vi "Validate Number.vi"(8 "error in (no error)":errorcluster, 11 "Number":i32 caption="Number to Validate") -> (0 "error out":errorcluster, 2 "Valid?":bool)   [LabVIEW 2017]
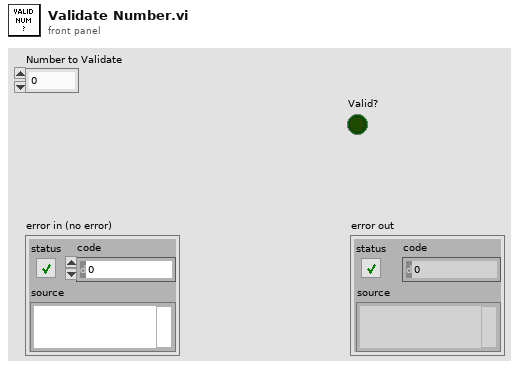
[diagram p1: front panel]
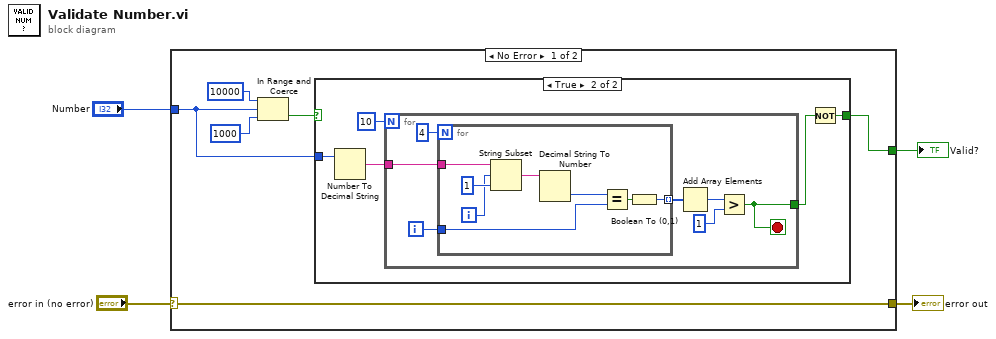
[diagram p0: block diagram]
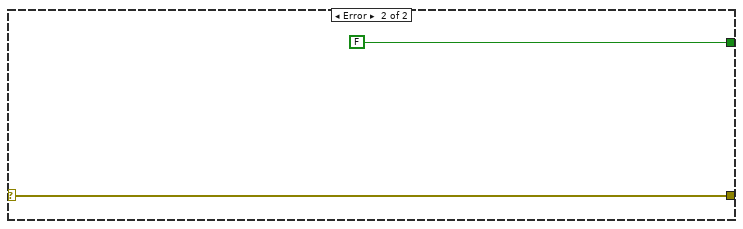
[diagram p3: hidden frame]
diagram:
  n1 = case shown="No Error" "error in (no error)" {
    selector: "error in (no error)" -> [w10 w33]
    tunnel: [w10 w33] -> w3
    tunnel: [w5 FALSE] -> w2
    tunnel: "Number" -> [w7 _]
    frame No Error {
      n2 = In Range and Coerce(upper limit=10000, x=w7, lower limit=1000) -> (In Range?=w6:bool)  [unwired: 1 out]
      n3 = case shown="True" w6 {
        selector: w6 -> [w11 _]
        tunnel: w7 -> [_ w16]
        tunnel: [w11 w12] -> w5
        frame False {
        }
        frame True {
          n4 = Number To Decimal String(number=w16) -> (decimal integer string=w15:string)  [unwired: 1 in]
          n5 = for {
            N: 10 -> [_]
            tunnel: w15 -> [w18]
            tunnel: [w19] -> w13
            i -> [w17]
            stop <- w19 stop-if-true
            n6 = for {
              N: 4 -> [_]
              tunnel: w17 -> [w24]
              tunnel: [w30] -> w22 mode=indexing
              tunnel: w18 -> [w27]
              i -> [w26]
              n7 = String Subset(string=w27, offset (0)=w26, length (rest)=1 ("length (rest)")) -> (substring=w28:string)
              n8 = Decimal String To Number(string=w28) -> (number=w25:i32)  [unwired: 2 in, 1 out]
              n9 = Equal?(x=w25, y=w24) -> (x = y?=w31:bool)
              n10 = Boolean To (0,1)(Boolean=w31) -> (0, 1=w30:i16)
            }
            n11 = Add Array Elements(numeric array=w22) -> (sum=w21:i16)
            n12 = Greater?(x=w21, y=i16 1) -> (0:w19:bool)
          }
          n13 = Not(x=w13) -> (.not. x?=w12:bool)
        }
      }
    }
    frame Error {
    }
  }
  "error out" <- w3
  "Valid?" <- w2
